vi "Billede_1_send.vi"() -> ()   [LabVIEW 2018]
uses:
  <vilib>/myRIO/Instrument Drivers/Onboard IO/UART/typedef/VISA Configuration.ctl
  <vilib>/Instr/_visa.llb/VISA Configure Serial Port (Instr).vi
  <vilib>/myRIO/Express VI/Onboard IO/UART/UART Express VI.xnode
  <vilib>/myRIO/Instrument Drivers/Onboard IO/UART/UART.lvlib
panel:
  out "length":i32
  out "spreadsheet string":string
  out "Intensity Graph 4":u8[][](graph)
  out "array":u8[][](array[numeric])
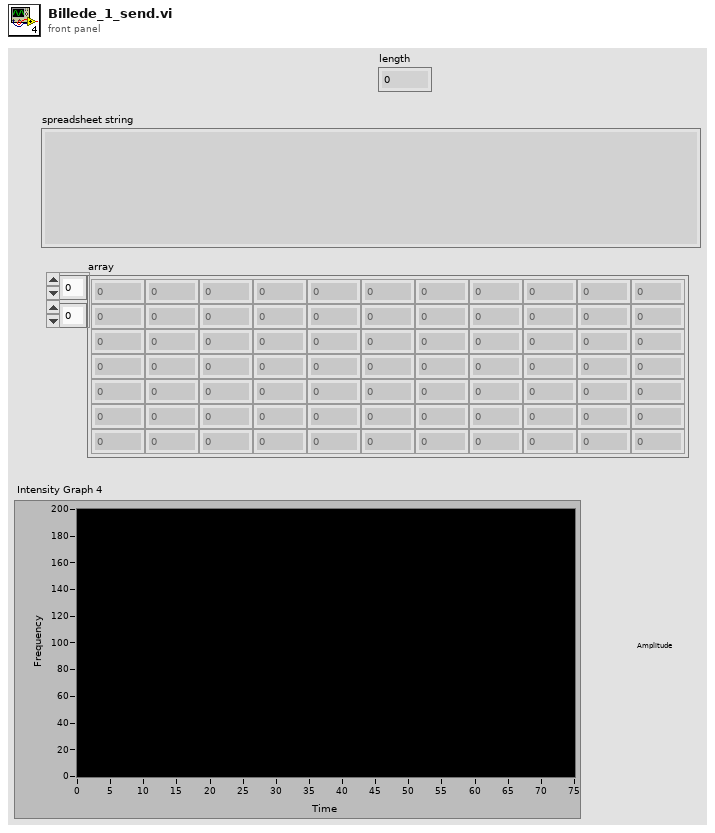
[diagram p1: front panel]
types:
  T1 = typedef "UART.lvlib/VISA Configuration.ctl" = cluster{"baud rate (9600)":u32, "data bits (8)":u16, "parity (0:none)":enum16{"None", "Odd", "Even", "Mark", "Space"}, "stop bits (10: 1 bit)":u16, "flow control (0:none)":u16, "termination char\n(0xA = '\\n' = LF) ":u8, "Enable Termination\nChar (T)":bool, "timeout (10sec)":u32}
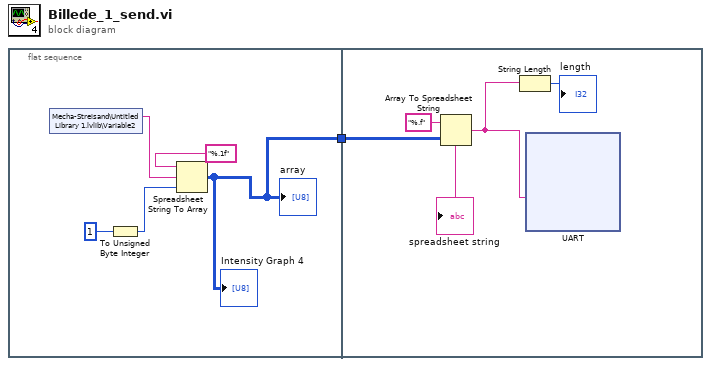
[diagram p0: block diagram]
diagram:
  n1 = flat-sequence {
    tunnel: [w2] -> w1
    tunnel: w1 -> [w9]
    frame #0 {
      n2 = shared-variable "Mecha-Streisand\\Untitled Library 1.lvlib\\Variable2"() -> (w3:string)  [unwired: 1 in, 1 out]
      n3 = To Unsigned Byte Integer(number=u8 1) -> (unsigned 8bit integer=w5:u8)
      n4 = Spreadsheet String To Array(format string="%.1f", spreadsheet string=w3, array type (2D Dbl)=w5) -> (array=w2:u8[][])  [unwired: 1 in]
      "array" <- w2
      "Intensity Graph 4" <- w2
    }
    frame #1 {
      n5 = Array To Spreadsheet String(array=w9, 3:"%.f" ("format string")) -> (spreadsheet string=w8:string)  [unwired: 1 in]
      "spreadsheet string" <- w8
      n6 = String Length(string=w8) -> (length=→"length":i32)
      n7 = xnode "UART"("Characters to Write"=w8) -> ()  [unwired: 1 in, 2 out]
    }
  }
